vi "ProgMon.ProgMon Core.vi"(9 "Ref CtrlEst":refnum<vi>, 11 "Ref CtrlComp":refnum<vi>) -> ()   [LabVIEW 2024, in "EQMF.lvlib" / "Status Utils.lvlib"]
uses:
  Status Utils.lvlib
  Queues/Q.Element.ctl
  Queues/Queue Utils.lvlib
panel:
  out "Value":dbl
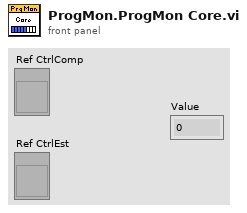
[diagram p1: front panel]
types:
  T1 = typedef "EQMF.lvlib/Queue Utils.lvlib/Q.Element.ctl" = cluster{"Cmd":string, "Sub":string, "Data1":variant, "Data2":variant}
  T2 = cluster{"Start":timestamp, "EstComp":timestamp, "Qt":i32, "Remaining(s)":dbl, "Ref CtrlComp":refnum<vi>, "Ref CtrlEst":refnum<vi>, "SuspendTime":timestamp}
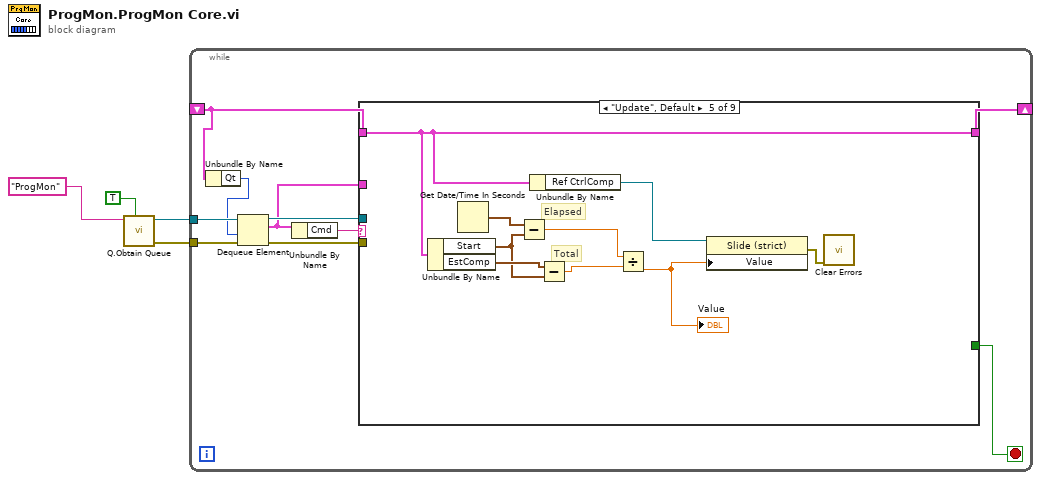
[diagram p0: block diagram]
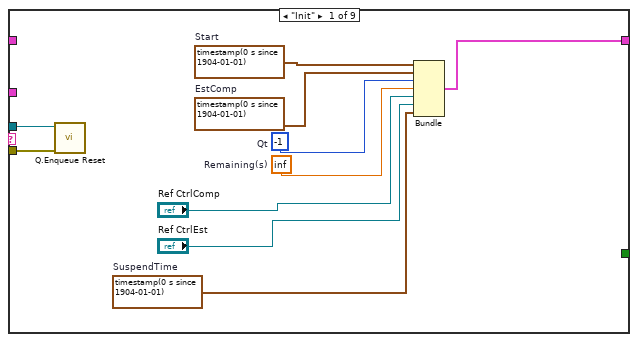
[diagram p2: hidden frame]
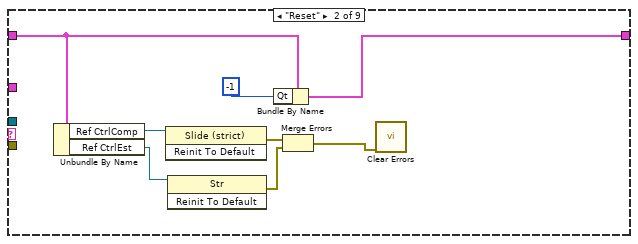
[diagram p3: hidden frame]
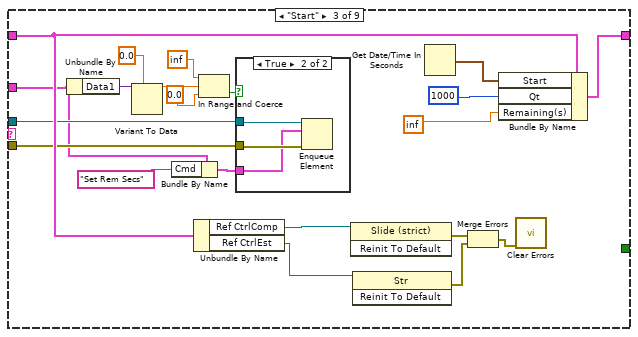
[diagram p4: hidden frame]
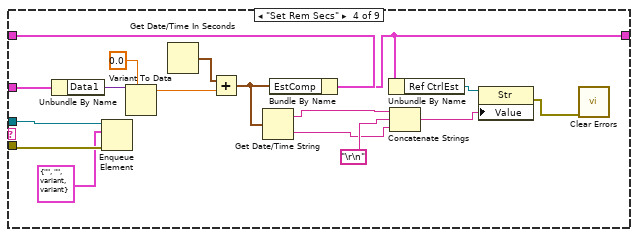
[diagram p6: hidden frame]
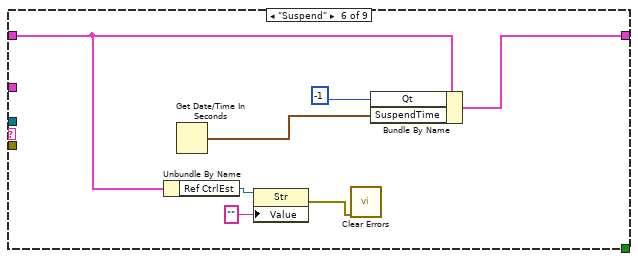
[diagram p7: hidden frame]
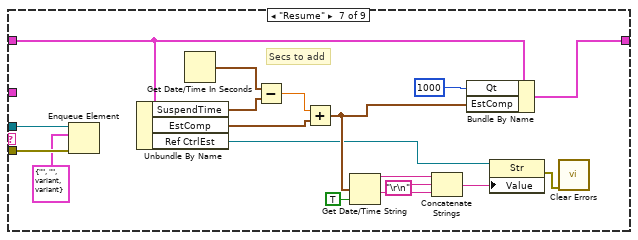
[diagram p8: hidden frame]
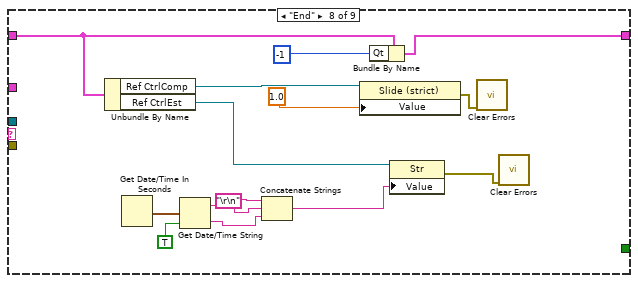
[diagram p9: hidden frame]
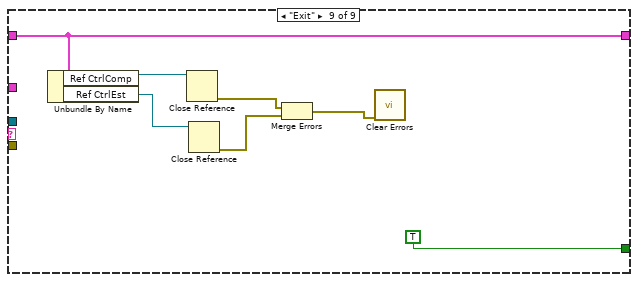
[diagram p10: hidden frame]
diagram:
  n1 = call "Q.Obtain Queue.vi"("Enqueue Init"=TRUE, "Q Name"="ProgMon" ("name (unnamed)")) -> ("error out"=w3:errorcluster, "Q Out"=w4:refnum<queue>)  [unwired: 7 in, 1 out]
  n2 = while {
    tunnel: w4 -> [w14]
    tunnel: w3 -> [w13]
    shift-right: [w7] -> _
    shift-left: _ -> [w6]
    stop <- w8 stop-if-true
    n3 = Unbundle By Name(w6) -> ("Qt"=w5:i32)
    n4 = Dequeue Element(queue=w14, timeout in ms (-1)=w5, error in (no error)=w13) -> (queue out=w12:refnum<queue>, element=w9:T1, error out=w10:errorcluster)  [unwired: 1 out]
    n5 = Unbundle By Name(w9) -> ("Cmd"=w11:string)
    n6 = case shown="\"Update\", Default" w11 {
      tunnel: w12 -> [w17 _ w38 w69 _ _ w93 _ _]
      tunnel: w10 -> [w16 _ w37 w68 _ _ w92 _ _]
      tunnel: w9 -> [_ _ w34 w72 _ _ _ _ _]
      tunnel: w6 -> [_ w30 w45 w73 w77 w84 w105 w111 w127]
      tunnel: [_ _ _ _ _ _ _ _ TRUE] -> w8
      tunnel: [w23 w31 w52 w60 w77 w87 w106 w110 w127] -> w7
      frame "Init" {
        w15 = timestamp(0 s since 1904-01-01)  # SuspendTime
        w20 = timestamp(0 s since 1904-01-01)  # EstComp
        w22 = inf  # Remaining(s)
        w21 = -1  # Qt
        w24 = timestamp(0 s since 1904-01-01)  # Start
        n7 = call "Q.Enqueue Reset.vi"("Error In"=w16, "Q In"=w17) -> ()  [unwired: 8 in, 2 out]
        n8 = Bundle("Start"=w24, "EstComp"=w20, "Qt"=w21, "Remaining(s)"=w22, "Ref CtrlComp"="Ref CtrlComp", "Ref CtrlEst"="Ref CtrlEst", "SuspendTime"=w15) -> (w23:T2)  [unwired: 1 in]
      }
      frame "Reset" {
        n9 = Unbundle By Name(w30) -> ("Ref CtrlComp"=w29:refnum<vi>, "Ref CtrlEst"=w28:refnum<vi>)
        n10 = invoke on="Invoke Node" class="Slide (strict)" method="Reinit To Default"(reference=w29) -> (error out=w27:errorcluster)  [unwired: 2 in, 2 out]
        n11 = invoke on="Invoke Node" class="Str" method="Reinit To Default"(reference=w28) -> (error out=w26:errorcluster)  [unwired: 2 in, 2 out]
        n12 = Bundle By Name(cluster=w30, "Qt"=-1) -> (w31:T2)
        n13 = Merge Errors(w27, w26) -> (w25:errorcluster)
        n14 = call <vilib>:"Clear Errors.vi"("error in (no error)"=w25) -> ()  [unwired: 5 in, 2 out]
      }
      frame "Start" {
        n15 = Unbundle By Name(w34) -> ("Data1"=w44:variant)
        n16 = Variant To Data(type=0.0, Variant=w44) -> (data=w39:dbl)  [unwired: 1 in, 1 out]
        n17 = Bundle By Name(cluster=w34, "Cmd"="Set Rem Secs") -> (w33:T1)
        n18 = Unbundle By Name(w45) -> ("Ref CtrlComp"=w50:refnum<vi>, "Ref CtrlEst"=w49:refnum<vi>)
        n19 = In Range and Coerce(upper limit=inf ("lower limit"), x=w39, lower limit=0.0) -> (In Range?=w36:bool)  [unwired: 1 out]
        n20 = case shown="True" w36 {
          tunnel: w38 -> [_ w56]
          tunnel: w37 -> [_ w55]
          tunnel: w33 -> [_ w54]
          frame False {
          }
          frame True {
            n21 = Enqueue Element(queue=w56, element=w54, error in (no error)=w55) -> ()  [unwired: 1 in, 3 out]
          }
        }
        n22 = invoke on="Invoke Node" class="Slide (strict)" method="Reinit To Default"(reference=w50) -> (error out=w48:errorcluster)  [unwired: 2 in, 2 out]
        n23 = invoke on="Invoke Node" class="Str" method="Reinit To Default"(reference=w49) -> (error out=w47:errorcluster)  [unwired: 2 in, 2 out]
        n24 = Get Date/Time In Seconds() -> (seconds since 1Jan1904=w51:timestamp)
        n25 = Merge Errors(w48, w47) -> (w46:errorcluster)
        n26 = Bundle By Name(cluster=w45, "Start"=w51, "Qt"=1000, "Remaining(s)"=inf) -> (w52:T2)
        n27 = call <vilib>:"Clear Errors.vi"("error in (no error)"=w46) -> ()  [unwired: 5 in, 2 out]
      }
      frame "Set Rem Secs" {
        n28 = Unbundle By Name(w72) -> ("Data1"=w71:variant)
        n29 = Enqueue Element(queue=w69, element=T1 {"Cmd"="", "Sub"="", "Data1"=variant, "Data2"=variant} ("MainQ.Element"), error in (no error)=w68) -> ()  [unwired: 1 in, 3 out]
        n30 = Variant To Data(type=0.0, Variant=w71) -> (data=w65:dbl)  [unwired: 1 in, 1 out]
        n31 = Get Date/Time In Seconds() -> (seconds since 1Jan1904=w66:timestamp)
        n32 = Add(x=w66, y=w65) -> (x+y=w61:timestamp)
        n33 = Get Date/Time String(seconds (now)=w61) -> (date string=w63:string, time string=w62:string)  [unwired: 2 in]
        n34 = Bundle By Name(cluster=w73, "EstComp"=w61) -> (w60:T2)
        n35 = Unbundle By Name(w60) -> ("Ref CtrlEst"=w59:refnum<vi>)
        n36 = Concatenate Strings(w63, "\r\n", w62) -> (w58:string)
        n37 = property class="Str"(reference=w59, "Value"=w58) -> (error out=w57:errorcluster)  [unwired: 1 in, 1 out]
        n38 = call <vilib>:"Clear Errors.vi"("error in (no error)"=w57) -> ()  [unwired: 5 in, 2 out]
      }
      frame "Update", Default {
        # "Total"
        # "Elapsed"
        n39 = Unbundle By Name(w77) -> ("Start"=w80:timestamp, "EstComp"=w81:timestamp)
        n40 = Get Date/Time In Seconds() -> (seconds since 1Jan1904=w82:timestamp)
        n41 = Subtract(x=w82, y=w80) -> (x-y=w79:dbl)
        n42 = Unbundle By Name(w77) -> ("Ref CtrlComp"=w76:refnum<vi>)
        n43 = Subtract(x=w81, y=w80) -> (x-y=w78:dbl)
        n44 = Divide(x=w79, y=w78) -> (x/y=w74:dbl)
        "Value" <- w74
        n45 = property class="Slide (strict)"(reference=w76, "Value"=w74) -> (error out=w75:errorcluster)  [unwired: 1 in, 1 out]
        n46 = call <vilib>:"Clear Errors.vi"("error in (no error)"=w75) -> ()  [unwired: 5 in, 2 out]
      }
      frame "Suspend" {
        n47 = Unbundle By Name(w84) -> ("Ref CtrlEst"=w85:refnum<vi>)
        n48 = Get Date/Time In Seconds() -> (seconds since 1Jan1904=w89:timestamp)
        n49 = property class="Str"(reference=w85, "Value"="") -> (error out=w83:errorcluster)  [unwired: 1 in, 1 out]
        n50 = call <vilib>:"Clear Errors.vi"("error in (no error)"=w83) -> ()  [unwired: 5 in, 2 out]
        n51 = Bundle By Name(cluster=w84, "Qt"=-1, "SuspendTime"=w89) -> (w87:T2)
      }
      frame "Resume" {
        # "Secs to add"
        n52 = Enqueue Element(queue=w93, element=T1 {"Cmd"="", "Sub"="", "Data1"=variant, "Data2"=variant} ("MainQ.Element"), error in (no error)=w92) -> ()  [unwired: 1 in, 3 out]
        n53 = Unbundle By Name(w105) -> ("SuspendTime"=w103:timestamp, "EstComp"=w101:timestamp, "Ref CtrlEst"=w95:refnum<vi>)
        n54 = Get Date/Time In Seconds() -> (seconds since 1Jan1904=w104:timestamp)
        n55 = Subtract(x=w104, y=w103) -> (x-y=w102:dbl)
        n56 = Add(x=w102, y=w101) -> (x+y=w97:timestamp)
        n57 = Get Date/Time String(seconds (now)=w97, want seconds? (F)=TRUE) -> (date string=w99:string, time string=w98:string)  [unwired: 1 in]
        n58 = Concatenate Strings(w99, "\r\n", w98) -> (w96:string)
        n59 = Bundle By Name(cluster=w105, "Qt"=1000, "EstComp"=w97) -> (w106:T2)
        n60 = property class="Str"(reference=w95, "Value"=w96) -> (error out=w94:errorcluster)  [unwired: 1 in, 1 out]
        n61 = call <vilib>:"Clear Errors.vi"("error in (no error)"=w94) -> ()  [unwired: 5 in, 2 out]
      }
      frame "End" {
        n62 = Unbundle By Name(w111) -> ("Ref CtrlComp"=w121:refnum<vi>, "Ref CtrlEst"=w114:refnum<vi>)
        n63 = Get Date/Time In Seconds() -> (seconds since 1Jan1904=w116:timestamp)
        n64 = Get Date/Time String(seconds (now)=w116, want seconds? (F)=TRUE) -> (date string=w118:string, time string=w117:string)  [unwired: 1 in]
        n65 = Concatenate Strings(w118, "\r\n", w117) -> (w113:string)
        n66 = property class="Slide (strict)"(reference=w121, "Value"=1.0) -> (error out=w120:errorcluster)  [unwired: 1 in, 1 out]
        n67 = Bundle By Name(cluster=w111, "Qt"=-1) -> (w110:T2)
        n68 = property class="Str"(reference=w114, "Value"=w113) -> (error out=w108:errorcluster)  [unwired: 1 in, 1 out]
        n69 = call <vilib>:"Clear Errors.vi"("error in (no error)"=w120) -> ()  [unwired: 5 in, 2 out]
        n70 = call <vilib>:"Clear Errors.vi"("error in (no error)"=w108) -> ()  [unwired: 5 in, 2 out]
      }
      frame "Exit" {
        n71 = Unbundle By Name(w127) -> ("Ref CtrlComp"=w126:refnum<vi>, "Ref CtrlEst"=w125:refnum<vi>)
        n72 = Close Reference(reference=w126) -> (error out=w123:errorcluster)  [unwired: 1 in]
        n73 = Close Reference(reference=w125) -> (error out=w122:errorcluster)  [unwired: 1 in]
        n74 = Merge Errors(w123, w122) -> (w124:errorcluster)
        n75 = call <vilib>:"Clear Errors.vi"("error in (no error)"=w124) -> ()  [unwired: 5 in, 2 out]
      }
    }
  }
